vi "Initialize Default Value Tree.vi"(11 "UI Data in":refnum<class "Settings UI.lvclass">) -> (2 "Items to Add":T1(array[cluster]), 3 "UI Data out":refnum<class "Settings UI.lvclass">)   [LabVIEW 2020, in "Output Sequencer.lvlib" / "Settings UI.lvclass"]
uses:
  Settings UI.lvclass
  Types/Tree Index Enum.ctl
  Settings UI.lvclass/Settings UI.ctl
  Globals/Global Tree Data.vi
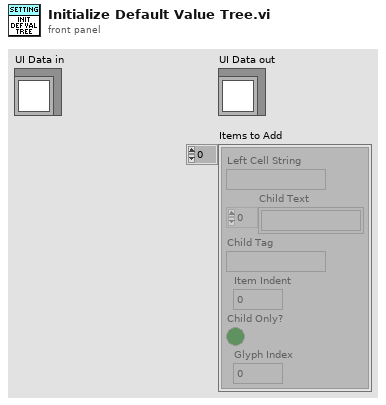
[diagram p1: front panel]
types:
  T1 = cluster{"Left Cell String":string, "Child Text":string[], "Child Tag":string, "Item Indent":i32, "Child Only?":bool, "Glyph Index":i32}[]
  T2 = typedef "Output Sequencer.lvlib/Settings UI.lvclass/Tree Index Enum.ctl" = enum16{"General Settings", "Num Steps", "Num Analog", "Num Digital", "Show Confirmation", "Interp Priority", "Adv Timing", "Enable Conditions", "Seq Execution", "Reset Test Start", "Only When Test", "Delay After Test", "Start condition", "Re-triggering", "Stop condition", "Stop After Cycles", "Stop Values", "Default Values", "Default Analog", "Default Digital", "Steps", "Step #", "Description", "Precondition", "Duration", "Mode", "Delay Between Vals", "Analog Values", "Digital Values", "Postcondition", "On True", "On False"}
  T3 = cluster{"Left Cell String":string, "Child Text":string[], "Child Tag":string, "Item Indent":i32, "Child Only?":bool, "Glyph Index":i32}
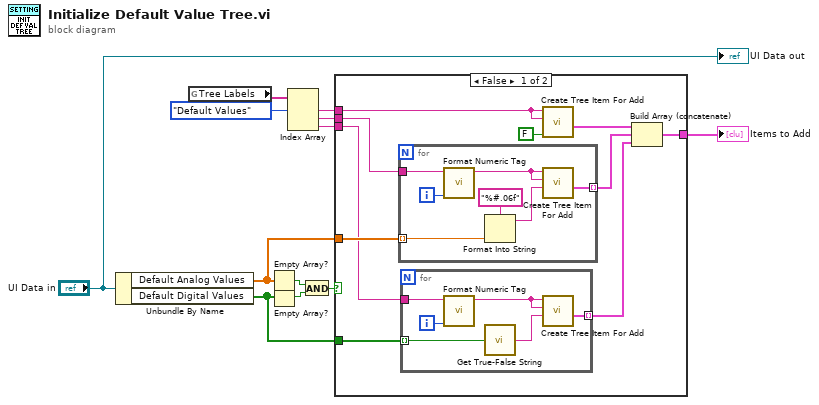
[diagram p0: block diagram]
diagram:
  n1 = Unbundle By Name("UI Data in") -> ("Default Analog Values"=w3:dbl[], "Default Digital Values"=w2:bool[])
  n2 = global read "Global Tree Data.vi" "Tree Labels"() -> (w11:string[])
  n3 = Empty Array?(array=w3) -> (empty?=w8:bool)
  n4 = Empty Array?(array=w2) -> (empty?=w7:bool)
  n5 = Index Array(array=w11, index #1=Tree_Index_Enum."Default Values" ("Tree Index Enum")) -> (element #1=w10:string, element #2=w9:string, element #3=w6:string)  [unwired: 2 in]
  n6 = And(x=w8, y=w7) -> (x .and. y?=w12:bool)
  n7 = case shown="False" w12 {
    tunnel: w10 -> [w18 _]
    tunnel: w9 -> [w22 _]
    tunnel: w3 -> [w21 _]
    tunnel: w6 -> [w17 _]
    tunnel: w2 -> [w16 _]
    tunnel: [w14 _] -> w5
    frame False {
      n8 = for {
        tunnel: w22 -> [w30]
        tunnel: w21 -> [w34] mode=indexing
        tunnel: [w33] -> w19 mode=indexing
        i -> [w29]
        n9 = call "Format Numeric Tag.vi"("Number"=w29, "Tree label"=w30) -> ("Tag"=w31:string)  [unwired: 9 in]
        n10 = Format Into String(format string="%#.06f", w34) -> (resulting string=w32:string)  [unwired: 2 in, 1 out]
        n11 = call "Create Tree Item For Add.vi"("Child Text"=w32, "Left Cell String"=w31, "Child Tag in"=w31) -> ("Item"=w33:T3)  [unwired: 7 in, 1 out]
      }
      n12 = for {
        tunnel: w17 -> [w25]
        tunnel: w16 -> [w27] mode=indexing
        tunnel: [w28] -> w15 mode=indexing
        i -> [w24]
        n13 = call "Format Numeric Tag.vi"("Number"=w24, "Tree label"=w25) -> ("Tag"=w23:string)  [unwired: 9 in]
        n14 = call "Get True-False String.vi"("Input"=w27) -> ("True/False String"=w26:string)
        n15 = call "Create Tree Item For Add.vi"("Child Text"=w26, "Left Cell String"=w23, "Child Tag in"=w23) -> ("Item"=w28:T3)  [unwired: 7 in, 1 out]
      }
      n16 = call "Create Tree Item For Add.vi"("Child Only? (true)"=FALSE ("Child Only?"), "Left Cell String"=w18, "Child Tag in"=w18) -> ("Item"=w20:T3)  [unwired: 7 in, 1 out]
      n17 = Build Array (concatenate)(w20, w19, w15) -> (w14:T1)
    }
    frame True {
    }
  }
  "Items to Add" <- w5
  "UI Data out" <- "UI Data in"
